vi "StringSize.vi"() -> ()   [LabVIEW 2019]
panel:
  out "length":i32
  in  "a":string="Pomogrenate"
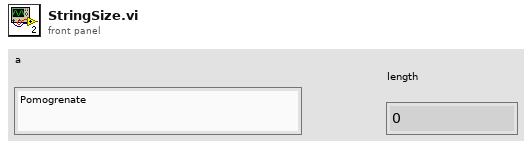
[diagram p1: front panel]
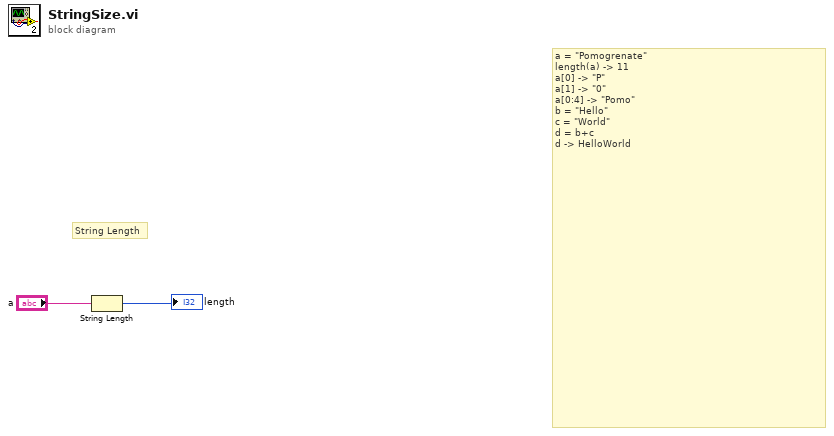
[diagram p0: block diagram]
diagram:
  # "String Length"
  # "a = \"Pomogrenate\"\nlength(a) -> 11\na[0] -> \"P\"\na[1] -> \"0\"\na[0:4] -> \"Pomo\"\nb = \"Hello\"\nc = \"World\"\nd = b+c\nd -> HelloWorld"
  n1 = String Length(string="a") -> (length=→"length":i32)
